vi "Guitar Subvi.vi"(0 "error out":errorcluster, 1 "Image Dst Out":T1, 2 "Blue Guitar 2":T2={"Global Rectangle"=[569, 290, 594, 372], "Contours"=[{"ID"=enum."External", "Type"=2, "Coordinates"=[593, 371, 569, 290]}]} {"Contours"."Type" items=["No Selection", "Point", "Line", "Rectangle", "Oval", "Polygon", "Freehand Region", "Annulus", "Unused2", "Unused3", "Broken Line", "Freehand Line", "Rotated Rectangle"]}, 3 "Yellow Guitar 2":T2={"Global Rectangle"=[546, 282, 563, 376], "Contours"=[{"ID"=enum."External", "Type"=2, "Coordinates"=[562, 375, 546, 282]}]} {"Contours"."Type" items=["No Selection", "Point", "Line", "Rectangle", "Oval", "Polygon", "Freehand Region", "Annulus", "Unused2", "Unused3", "Broken Line", "Freehand Line", "Rotated Rectangle"]}, 4 "Green Guitar 2":T2={"Global Rectangle"=[498, 284, 505, 376], "Contours"=[{"ID"=enum."External", "Type"=2, "Coordinates"=[498, 375, 504, 284]}]} {"Contours"."Type" items=["No Selection", "Point", "Line", "Rectangle", "Oval", "Polygon", "Freehand Region", "Annulus", "Unused2", "Unused3", "Broken Line", "Freehand Line", "Rotated Rectangle"]}, 5 "Red Guitar 2":T2={"Global Rectangle"=[526, 284, 530, 370], "Contours"=[{"ID"=enum."External", "Type"=2, "Coordinates"=[529, 369, 526, 284]}]} {"Contours"."Type" items=["No Selection", "Point", "Line", "Rectangle", "Oval", "Polygon", "Freehand Region", "Annulus", "Unused2", "Unused3", "Broken Line", "Freehand Line", "Rotated Rectangle"]}, 6 "Orange Guitar 2":T2={"Global Rectangle"=[587, 282, 628, 378], "Contours"=[{"ID"=enum."External", "Type"=2, "Coordinates"=[627, 377, 587, 282]}]} {"Contours"."Type" items=["No Selection", "Point", "Line", "Rectangle", "Oval", "Polygon", "Freehand Region", "Annulus", "Unused2", "Unused3", "Broken Line", "Freehand Line", "Rotated Rectangle"]}) -> (11 "Orange Guitar LED":bool, 13 "Red Guitar LED":bool, 15 "Green Guitar LED":bool, 23 "Blue Guitar LED":bool, 24 "Yellow Guitar LED":bool, 27 "error out 2":errorcluster)   [LabVIEW 2009]
uses:
  <vilib>/vision/Image Controls.llb/IMAQ Image.ctl
  <vilib>/Analysis/3filter.llb/Filter Passband Type.ctl
  <vilib>/Analysis/3filter.llb/Butterworth Filter (DBL).vi
  <vilib>/Analysis/NI_AALBase.lvlib
  <vilib>/vision/NI_Vision_Development_Module.lvlib
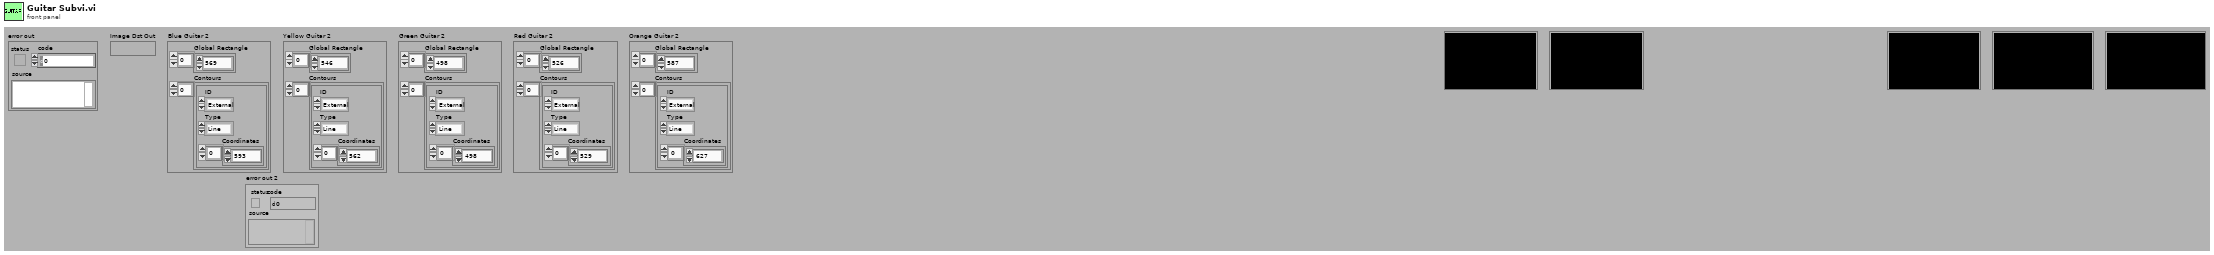
[diagram p1: front panel]
types:
  T1 = typedef "IMAQ Image.ctl" = refnum<image>
  T2 = cluster{"Global Rectangle":i32[], "Contours":cluster{"ID":enum32{"External", "Internal"}, "Type":u32, "Coordinates":i32[]}[]}
  T3 = typedef "NI_AALBase.lvlib/Filter Passband Type.ctl" = enum32{"Lowpass", "Highpass", "Bandpass", "Bandstop"}
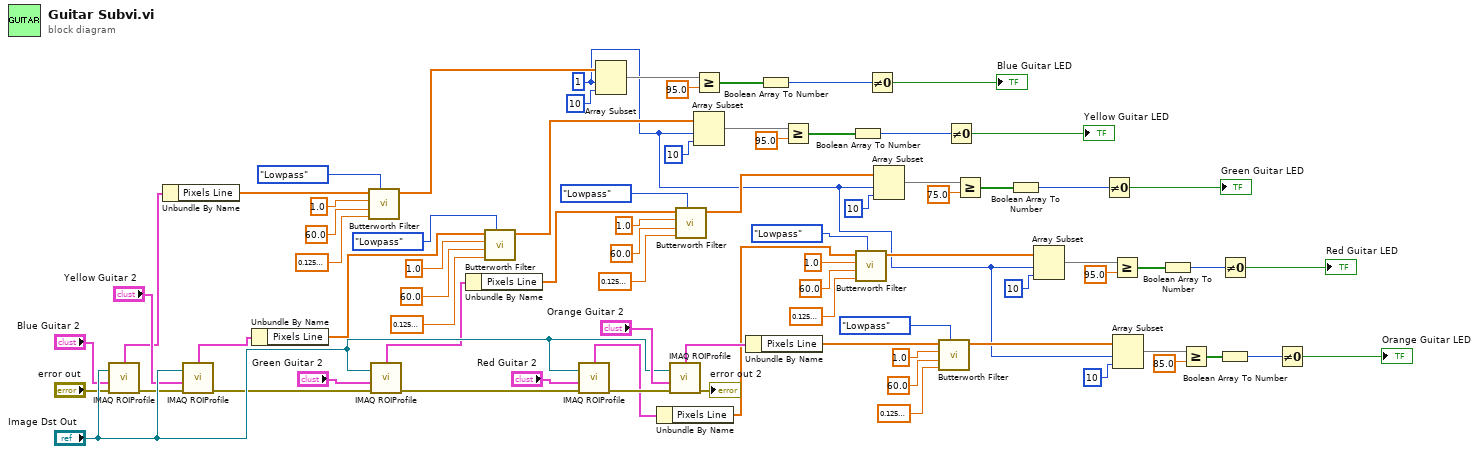
[diagram p0: block diagram]
diagram:
  w2 = 1 ("index")
  n1 = call "IMAQ ROIProfile"("error in (no error)"="error out", "ROI Descriptor"="Blue Guitar 2", "Image"="Image Dst Out") -> ("error out"=w43:errorcluster, "ROI Graph"=w42:cluster{"x0":sgl, "dx":sgl, "Pixels Line":sgl[]})  [unwired: 4 out]
  n2 = Unbundle By Name(w42) -> ("Pixels Line"=w63:sgl[])
  n3 = call "IMAQ ROIProfile"("error in (no error)"=w43, "ROI Descriptor"="Yellow Guitar 2", "Image"="Image Dst Out") -> ("error out"=w15:errorcluster, "ROI Graph"=w46:cluster{"x0":sgl, "dx":sgl, "Pixels Line":sgl[]})  [unwired: 4 out]
  n4 = Unbundle By Name(w46) -> ("Pixels Line"=w49:sgl[])
  n5 = call-poly <vilib>:"Butterworth Filter.vi"("filter type"=Filter_Passband_Type."Lowpass", "low cutoff freq: fl"=0.12500000000000006 ("low 3"), "high cutoff freq: fh"=60.0 ("high 14"), "sampling freq: fs"=1.0 ("sampling  9"), "X"=w63) -> ("Filtered X"=w29:dbl[])  [unwired: 3 in, 1 out]
  n6 = call "IMAQ ROIProfile"("error in (no error)"=w15, "ROI Descriptor"="Green Guitar 2", "Image"="Image Dst Out") -> ("error out"=w16:errorcluster, "ROI Graph"=w40:cluster{"x0":sgl, "dx":sgl, "Pixels Line":sgl[]})  [unwired: 4 out]
  n7 = Unbundle By Name(w40) -> ("Pixels Line"=w37:sgl[])
  n8 = call-poly <vilib>:"Butterworth Filter.vi"("filter type"=Filter_Passband_Type."Lowpass", "low cutoff freq: fl"=0.12500000000000006 ("low  12"), "high cutoff freq: fh"=60.0 ("high 13"), "sampling freq: fs"=1.0 ("sampling 12"), "X"=w49) -> ("Filtered X"=w45:dbl[])  [unwired: 3 in, 1 out]
  n9 = call "IMAQ ROIProfile"("error in (no error)"=w16, "ROI Descriptor"="Red Guitar 2", "Image"="Image Dst Out") -> ("error out"=w71:errorcluster, "ROI Graph"=w18:cluster{"x0":sgl, "dx":sgl, "Pixels Line":sgl[]})  [unwired: 4 out]
  n10 = Array Subset(array=w29, index=w2, length=10) -> (w58:dbl[])
  n11 = Unbundle By Name(w18) -> ("Pixels Line"=w21:sgl[])
  n12 = call "IMAQ ROIProfile"("error in (no error)"=w71, "ROI Descriptor"="Orange Guitar 2", "Image"="Image Dst Out") -> ("error out"=→"error out 2":errorcluster, "ROI Graph"=w72:cluster{"x0":sgl, "dx":sgl, "Pixels Line":sgl[]})  [unwired: 4 out]
  n13 = call-poly <vilib>:"Butterworth Filter.vi"("filter type"=Filter_Passband_Type."Lowpass", "low cutoff freq: fl"=0.12500000000000006 ("low  11"), "high cutoff freq: fh"=60.0 ("high 12"), "sampling freq: fs"=1.0 ("sampling 11"), "X"=w37) -> ("Filtered X"=w41:dbl[])  [unwired: 3 in, 1 out]
  n14 = Greater Or Equal?(x=w58, y=95.0) -> (x >= y?=w3:bool[])
  n15 = Array Subset(array=w45, index=w2, length=10) -> (w54:dbl[])
  n16 = Unbundle By Name(w72) -> ("Pixels Line"=w11:sgl[])
  n17 = Boolean Array To Number(Boolean array=w3) -> (number=w56:u32)
  n18 = Greater Or Equal?(x=w54, y=95.0) -> (x >= y?=w52:bool[])
  n19 = Boolean Array To Number(Boolean array=w52) -> (number=w51:u32)
  n20 = call-poly <vilib>:"Butterworth Filter.vi"("filter type"=Filter_Passband_Type."Lowpass", "low cutoff freq: fl"=0.12500000000000006 ("low  10"), "high cutoff freq: fh"=60.0 ("high 11"), "sampling freq: fs"=1.0 ("sampling 10"), "X"=w21) -> ("Filtered X"=w17:dbl[])  [unwired: 3 in, 1 out]
  n21 = Not Equal To 0?(x=w56) -> (x != 0?=→"Blue Guitar LED":bool)
  n22 = Array Subset(array=w41, index=w2, length=10) -> (w32:dbl[])
  n23 = call-poly <vilib>:"Butterworth Filter.vi"("filter type"=Filter_Passband_Type."Lowpass", "low cutoff freq: fl"=0.12500000000000006 ("low  9"), "high cutoff freq: fh"=60.0 ("high 10"), "sampling freq: fs"=1.0 ("sampling 9"), "X"=w11) -> ("Filtered X"=w14:dbl[])  [unwired: 3 in, 1 out]
  n24 = Not Equal To 0?(x=w51) -> (x != 0?=→"Yellow Guitar LED":bool)
  n25 = Greater Or Equal?(x=w32, y=75.0) -> (x >= y?=w34:bool[])
  n26 = Boolean Array To Number(Boolean array=w34) -> (number=w35:u32)
  n27 = Array Subset(array=w17, index=w2, length=10) -> (w26:dbl[])
  n28 = Not Equal To 0?(x=w35) -> (x != 0?=→"Green Guitar LED":bool)
  n29 = Greater Or Equal?(x=w26, y=95.0) -> (x >= y?=w24:bool[])
  n30 = Array Subset(array=w14, index=w2, length=10) -> (w6:dbl[])
  n31 = Boolean Array To Number(Boolean array=w24) -> (number=w23:u32)
  n32 = Greater Or Equal?(x=w6, y=85.0) -> (x >= y?=w8:bool[])
  n33 = Not Equal To 0?(x=w23) -> (x != 0?=→"Red Guitar LED":bool)
  n34 = Boolean Array To Number(Boolean array=w8) -> (number=w9:u32)
  n35 = Not Equal To 0?(x=w9) -> (x != 0?=→"Orange Guitar LED":bool)
